vi "Write Vertical Scrollbar Visibility.vi"(5 "Vertical Scrollbar Visibility":T1(ring), 9 "Pane in":refnum<class "Pane.lvclass">) -> (3 "Pane out":refnum<class "Pane.lvclass">)   [LabVIEW 2014, in "Pane.lvclass"]
uses:
  Pane.lvclass
  Pane.lvclass/Pane.ctl
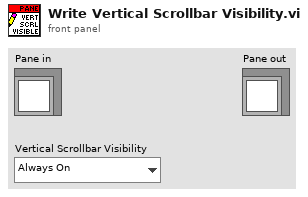
[diagram p1: front panel]
types:
  T1 = enum16{"Always On", "Always Off", "Off While Running"}
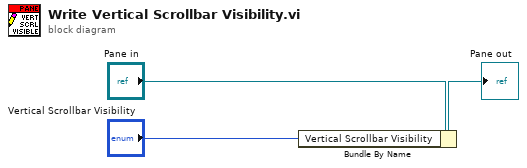
[diagram p0: block diagram]
diagram:
  n1 = Bundle By Name(cluster="Pane in", "Vertical Scrollbar Visibility"="Vertical Scrollbar Visibility") -> (→"Pane out":refnum<class "Pane.lvclass">)
